vi "Get Log - Last.vi"(0 "reference in":refnum<class "Result Logger.lvclass">, 5 "error in (no error)":errorcluster) -> (14 "reference out":refnum<class "Result Logger.lvclass">, 18 "Message":T1, 19 "error out":errorcluster)   [LabVIEW 2017, in "Result Logger.lvclass"]
uses:
  Result Logger.lvclass
  public/Message.ctl
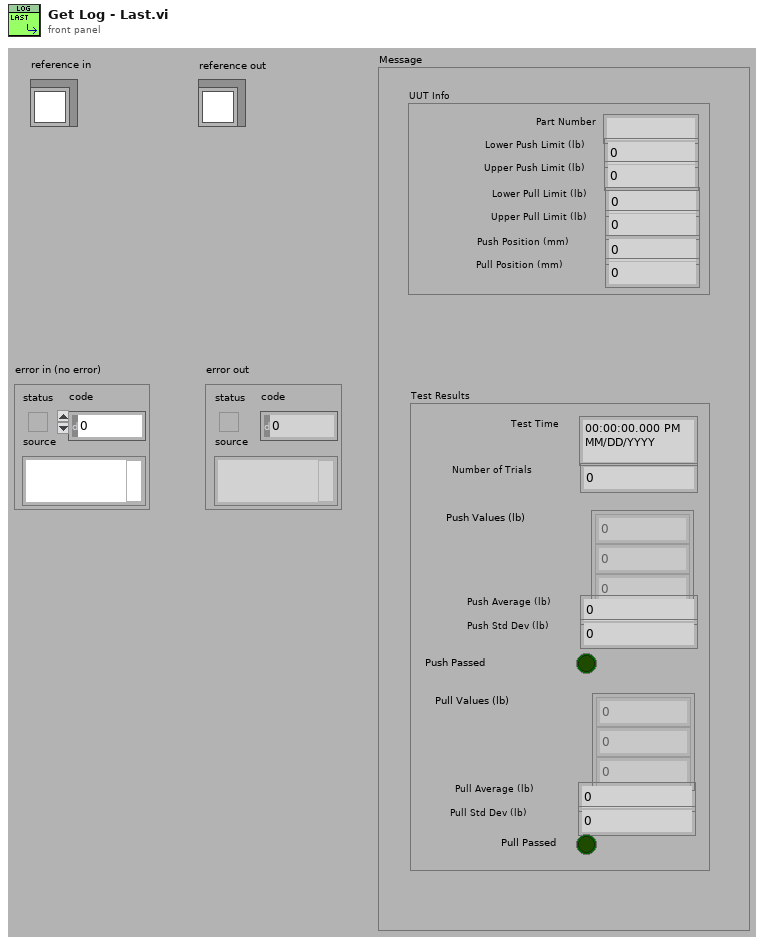
[diagram p1: front panel]
types:
  T1 = typedef "Result Logger.lvclass/Message.ctl" = cluster{"UUT Info":cluster{"Part Number":string, "Lower Push Limit (lb)":dbl, "Upper Push Limit (lb)":dbl, "Lower Pull Limit (lb)":dbl, "Upper Pull Limit (lb)":dbl, "Push Position (mm)":dbl, "Pull Position (mm)":dbl}, "Test Results":cluster{"Test Time":timestamp, "Number of Trials":u32, "Push Values (lb)":dbl[], "Push Average (lb)":dbl, "Push Std Dev (lb)":dbl, "Push Passed":bool, "Pull Values (lb)":dbl[], "Pull Average (lb)":dbl, "Pull Std Dev (lb)":dbl, "Pull Passed":bool}}
  T2 = typedef "Result Logger.lvclass/ObjectAttributes.ctl" = cluster{"Logger File Path":path, "Logger File Stream":refnum<file>, "Log Messages":T1[]}
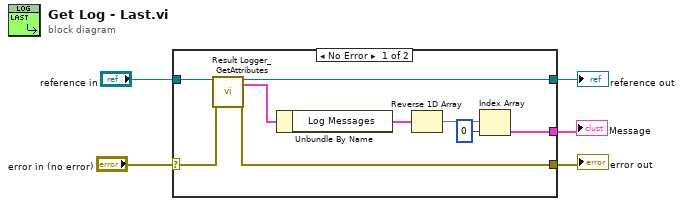
[diagram p0: block diagram]
diagram:
  n1 = case shown="No Error" "error in (no error)" {
    selector: "error in (no error)" -> [w14 w16]
    tunnel: [w13 w16] -> w4
    tunnel: [w11 w15] -> w2
    tunnel: "reference in" -> [w12 w15]
    tunnel: [w6 _] -> w1
    frame No Error {
      n2 = call "Result Logger_GetAttributes.vi"("reference in"=w12, "error in (no error)"=w14) -> ("reference out"=w11:refnum<class "Result Logger.lvclass">, "Data"=w7:T2, "error out"=w13:errorcluster)  [unwired: 14 in, 1 out]
      n3 = Unbundle By Name(w7) -> ("Log Messages"=w8:T1[])
      n4 = Reverse 1D Array(array=w8) -> (reversed array=w9:T1[])
      n5 = Index Array(array=w9, index=0) -> (element=w6:T1)
    }
    frame Error {
    }
  }
  "error out" <- w4
  "reference out" <- w2
  "Message" <- w1
